vi "GetPhase.vi"(10 "mag/phase":T1 items=["FRF", "rad phase unwrapped", "deg phase unwrapped", "rad phase wrapped", "deg phase wrapped", "White Plots", "MJ Map", "Real and Imaginary"], 11 "FRF in":cluster{dbl, "df":dbl, cdb[]}[](array[cluster])) -> (3 "Array":cluster{dbl, "df":dbl, dbl[]}[](array[cluster]))   [LabVIEW 2022 SP3]
uses:
  GraphType.ctl
  <vilib>/Analysis/NI_AALPro.lvlib
panel:
  out "Numeric":dbl
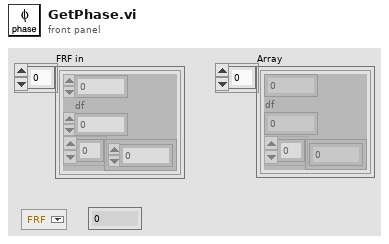
[diagram p1: front panel]
types:
  T1 = typedef "GraphType.ctl" = u16
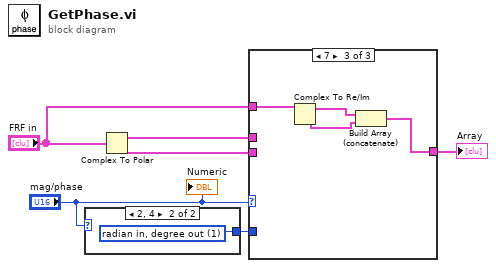
[diagram p0: block diagram]
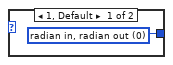
[diagram p2: hidden frame]
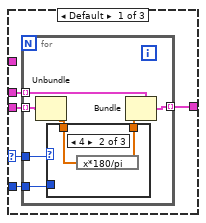
[diagram p3: hidden frame]
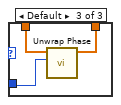
[diagram p5: hidden frame]
diagram:
  n1 = case shown="2, 4" "mag/phase" {
    tunnel: [w7 w8] -> w4
    frame 1, Default {
      w7 = 0 items=["radian in, radian out", "radian in, degree out", "degree in, degree out", "degree in, radian out"] ("phase unit")
    }
    frame 2, 4 {
      w8 = 1 items=["radian in, radian out", "radian in, degree out", "degree in, degree out", "degree in, radian out"] ("phase unit")
    }
  }
  n2 = Complex To Polar(r * e^(i*theta)="FRF in") -> (r=w3:cluster{dbl, "df":dbl, dbl[]}[], theta=w2:cluster{dbl, "df":dbl, dbl[]}[])
  n3 = case shown="7" "mag/phase" {
    selector: "mag/phase" -> [w11 _ _]
    tunnel: [w13 w27 w28] -> w6
    tunnel: w4 -> [w12 _ _]
    tunnel: w3 -> [w9 w27 _]
    tunnel: w2 -> [w10 _ _]
    tunnel: "FRF in" -> [_ _ w31]
    frame Default {
      n4 = for {
        tunnel: [w20] -> w13 mode=indexing
        tunnel: w12 -> [w18]
        tunnel: w11 -> [w16]
        tunnel: w10 -> [w15] mode=indexing
        tunnel: w9 -> [w14] mode=indexing
        n5 = Unbundle(w15) -> (w19:dbl[])  [unwired: 2 out]
        n6 = case shown="4" w16 {
          tunnel: w19 -> [w21 w23 w26]
          tunnel: w18 -> [_ _ w25]
          tunnel: [w21 w22 w24] -> w17
          frame 3 {
          }
          frame 4 {
            n7 = expression code="x*180/pi"(w23) -> (w22:dbl[])
          }
          frame Default {
            n8 = call <vilib>:"Unwrap Phase.vi"("phase unit"=w25, "Phase"=w26) -> ("Unwrapped Phase"=w24:dbl[])  [unwired: 8 in, 1 out]
          }
        }
        n9 = Bundle(cluster=w14, w17) -> (w20:cluster{dbl, "df":dbl, dbl[]})  [unwired: 2 in]
      }
    }
    frame 0, 6 {
    }
    frame 7 {
      n10 = Complex To Re/Im(x + iy=w31) -> (x=w30:cluster{dbl, "df":dbl, dbl[]}[], y=w29:cluster{dbl, "df":dbl, dbl[]}[])
      n11 = Build Array (concatenate)(w30, w29) -> (w28:cluster{dbl, "df":dbl, dbl[]}[])
    }
  }
  "Array" <- w6
  "Numeric" <- "mag/phase"
